vi "exit.vi"(8 "error in (no error)":errorcluster, 10 "model in":refnum<class "IModel.lvclass">, 11 "StandbyState in":refnum<class "StandbyState.lvclass">) -> (0 "error out":errorcluster, 2 "model out":refnum<class "IModel.lvclass">, 3 "StandbyState out":refnum<class "StandbyState.lvclass">)   [LabVIEW 2016, in "States.lvlib" / "StandbyState.lvclass"]
uses:
  StandbyState.lvclass
  IModel/IModel.lvclass
  Typedefs/CommandValue.ctl
  ts_sallv_exa/DataTypes/logevent_DetailedState.ctl
  ts_sallv_exa/DataTypes/logevent_SummaryState.ctl
  ComponentTemplateCore/ComponentModel/ComponentModel/InternalSignals/stop.vi
  ComponentTemplateCore/ComponentModel/ComponentModel/InternalSignals/InternalSignalsGlobals.lvlib
  Typedefs/EXATypedefs.lvlib
  ts_sallv_exa/SALLV_EXA.lvlib
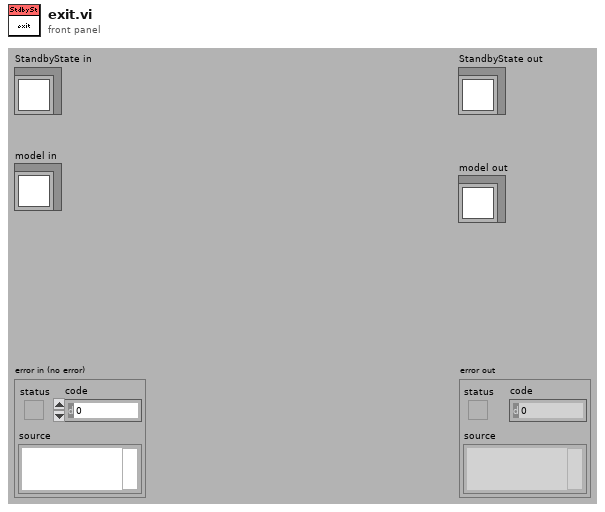
[diagram p1: front panel]
types:
  T1 = typedef "SALLV_EXA.lvlib/logevent_SummaryState.ctl" = cluster{"summaryState":enum16{"", "DisabledState", "EnabledState", "FaultState", "OfflineState", "StandbyState"}, "priority":i32}
  T2 = typedef "SALLV_EXA.lvlib/logevent_DetailedState.ctl" = cluster{"detailedState":enum16{"", "DisabledState", "EnabledState", "FaultState", "OfflineState", "StandbyState"}, "priority":i32}
  T3 = typedef "EXATypedefs.lvlib/CommandValue.ctl" = enum16{"Disable", "Enable", "Exit", "GoToStandby", "OnHeartbeat", "OnIncomingMessagingError", "OnInterrupt", "Start"}
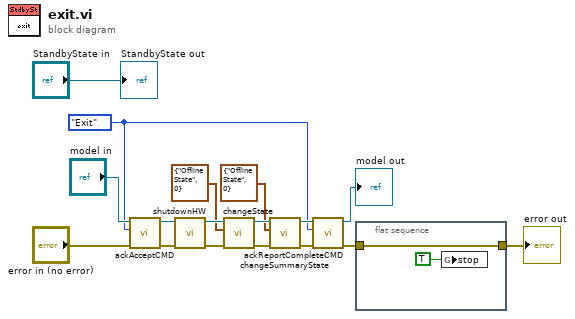
[diagram p0: block diagram]
diagram:
  w5 = CommandValue."Exit" ("CommandValue")
  n1 = call-dynamic "ackAcceptCMD.vi"("error in (no error)"="error in (no error)", "CommandValue"=w5, "IModel in"="model in") -> ("error out"=w8:errorcluster, "IModel out"=w9:refnum<class "IModel.lvclass">)  [unwired: 7 in]
  n2 = call-dynamic "shutdownHW.vi"("error in (no error)"=w8, "IModel in"=w9) -> ("error out"=w14:errorcluster, "IModel out"=w13:refnum<class "IModel.lvclass">)  [unwired: 8 in]
  n3 = call-dynamic "changeState.vi"("error in (no error)"=w14, "DetailedState"=T2 {"detailedState"=enum."OfflineState", "priority"=0} ("logevent_DetailedState"), "IModel in"=w13) -> ("error out"=w15:errorcluster, "IModel out"=w16:refnum<class "IModel.lvclass">)  [unwired: 7 in]
  n4 = call-dynamic "changeSummaryState.vi"("error in (no error)"=w15, "logevent_SummaryState"=T1 {"summaryState"=enum."OfflineState", "priority"=0}, "IModel in"=w16) -> ("error out"=w12:errorcluster, "IModel out"=w10:refnum<class "IModel.lvclass">)  [unwired: 7 in]
  n5 = call-dynamic "ackReportCompleteCMD.vi"("error in (no error)"=w12, "CommandValue"=w5, "IModel in"=w10) -> ("error out"=w3:errorcluster, "IModel out"=→"model out":refnum<class "IModel.lvclass">)  [unwired: 7 in]
  n6 = flat-sequence {
    tunnel: [w19] -> w4
    tunnel: w3 -> [w19]
    frame #0 {
      n7 = global write "stop.vi" "stop"(TRUE ("stop")) -> ()
    }
  }
  "error out" <- w4
  "StandbyState out" <- "StandbyState in"
